vi "arduino.vi"(8 "error in (no error)":errorcluster, 11 "VISA Refnum in":refnum<visa-resource-name>) -> (0 "error out":errorcluster, 2 "Waveform Chart":dbl[](graph), 3 "VISA Refnum in 2":refnum<visa-resource-name>)   [LabVIEW 2022 SP3]
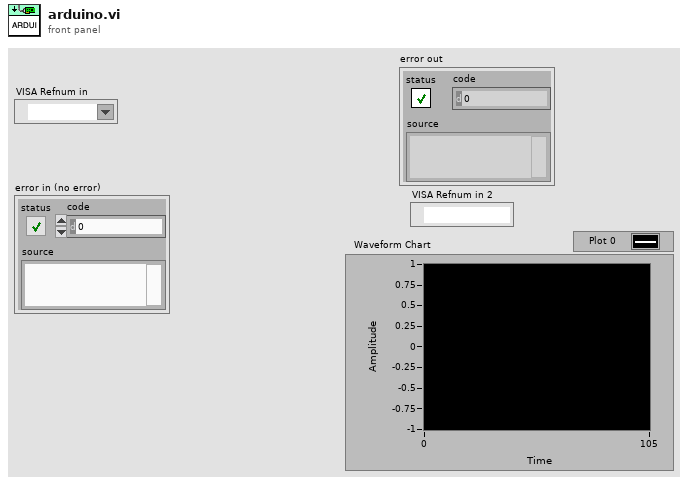
[diagram p1: front panel]
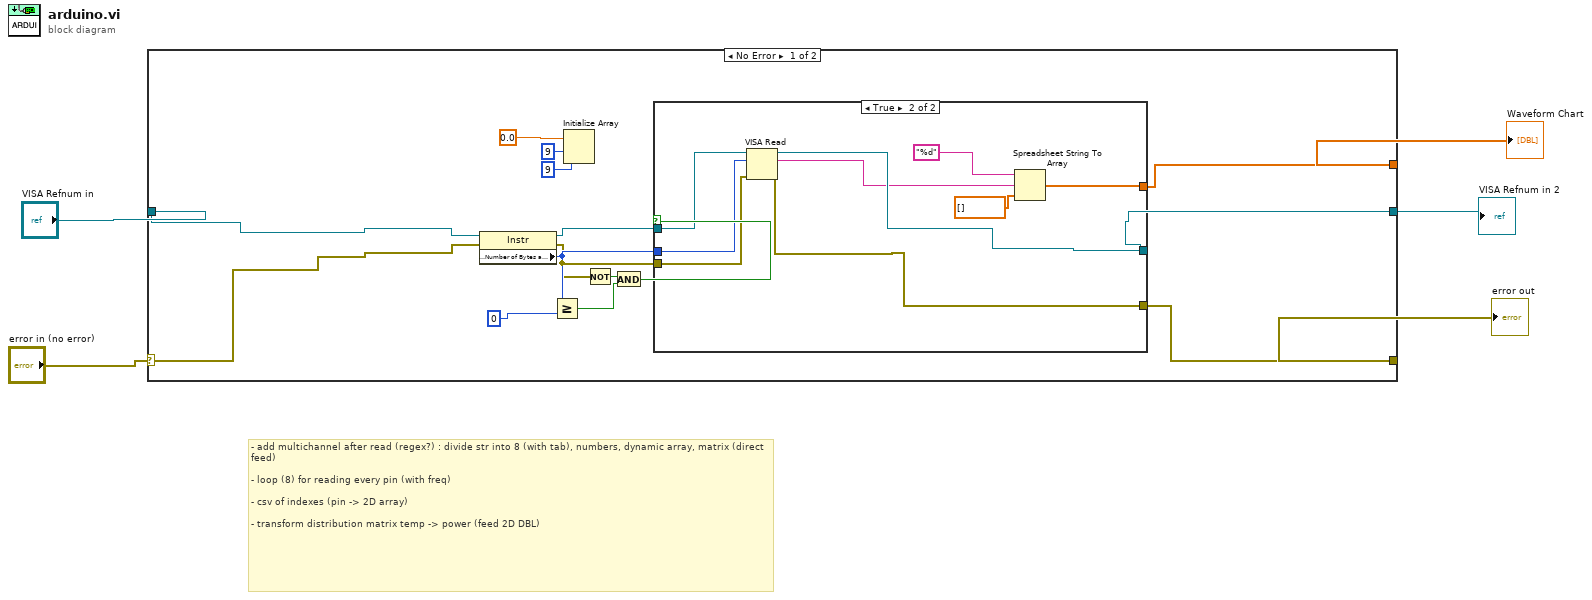
[diagram p0: block diagram]
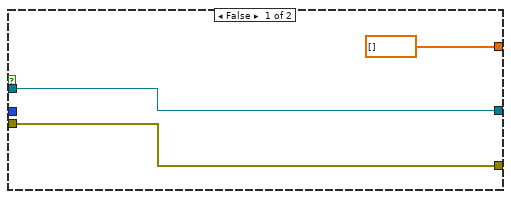
[diagram p2: hidden frame]
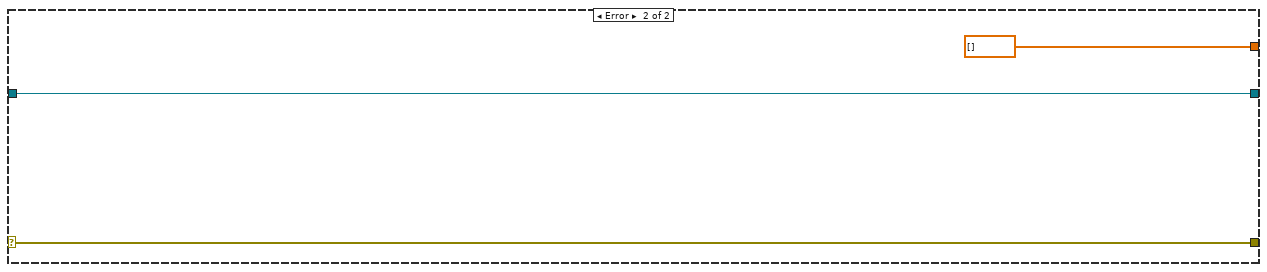
[diagram p3: hidden frame]
diagram:
  # "- add multichannel after read (regex?) : divide str into 8 (with tab), numbers, dynamic array, matrix (direct feed)\n\n- loop (8) for reading every pin (with freq)\n\n- csv of indexes (pin -> 2D array)\n\n- transform distribution matrix temp -> power (feed 2D DBL)"
  n1 = case shown="No Error" "error in (no error)" {
    selector: "error in (no error)" -> [w15 w35]
    tunnel: [w17 w35] -> w4
    tunnel: "VISA Refnum in" -> [w16 w34]
    tunnel: [w18 w34] -> w1
    tunnel: [w6 dbl[] [] ("Measurements")] -> w3
    frame No Error {
      n2 = property class="Instr"(reference=w16, error in=w15) -> (reference out=w20:refnum<visa-resource-name>, error out=w10:errorcluster, "Serial Settings:Number of Bytes at Serial Port"=w14:u32)
      n3 = Greater Or Equal?(x=w14, y=0) -> (x >= y?=w13:bool)
      n4 = Initialize Array(0.0 ("element"), 9 ("dimension size"), 9 ("dimension size")) -> ()  [unwired: 1 out]
      n5 = Not(x=w10) -> (.not. x?=w12:bool)
      n6 = And(x=w12, y=w13) -> (x .and. y?=w11:bool)
      n7 = case shown="True" w11 {
        tunnel: w20 -> [w23 w32]
        tunnel: w14 -> [_ w26]
        tunnel: [w23 w30] -> w18
        tunnel: [dbl[] [] ("Measurements") w24] -> w6
        tunnel: [w21 w29] -> w17
        tunnel: w10 -> [w21 w31]
        frame False {
        }
        frame True {
          n8 = VISA Read(VISA resource name=w32, byte count=w26, error in (no error)=w31) -> (VISA resource name out=w30:refnum<visa-resource-name>, read buffer=w27:string, error out=w29:errorcluster)  [unwired: 1 out]
          n9 = Spreadsheet String To Array(format string="%d", spreadsheet string=w27, array type (2D Dbl)=dbl[] []) -> (array=w24:dbl[])  [unwired: 1 in]
        }
      }
    }
    frame Error {
    }
  }
  "error out" <- w4
  "Waveform Chart" <- w3
  "VISA Refnum in 2" <- w1
